vi "LeerBD.vi"(8 "error in (no error)":errorcluster) -> (0 "error out":errorcluster, 2 "BD":T1={"niv_presion_son_ref"=97.0, "Incertidumbre"=["1", "1", "1", "1", "1", "1", "1", "1", "1", "1"], "Tol +"=["2,0", "1,5", "1,5", "1,4", "1,4", "1,1", "1,6", "1,6", "2,1", "3,5"], "Tol -"=["-2,0", "-1,5", "-1,5", "-1,4", "-1,4", "-1,1", "-1,6", "-1,6", "-2,1", "-3,5"], "Frecuencias(Hz)"=["95", "94", "94", "94", "96", "95", "94", "96", "95", "94"]}, 3 "Prueba05 out":refnum<class "Prueba05.lvclass">)   [LabVIEW 2019, in "Prueba05.lvclass"]
uses:
  Prueba05.lvclass
  BD.ctl
  Base de Datos/SQLiteConnector/SQLiteConnection.lvclass
  Base de Datos/Base de Datos.lvclass
panel:
  in  "Tipo Equipo":enum16{"Sonometro", "Calibrador", "Dosimetro"}(ring)
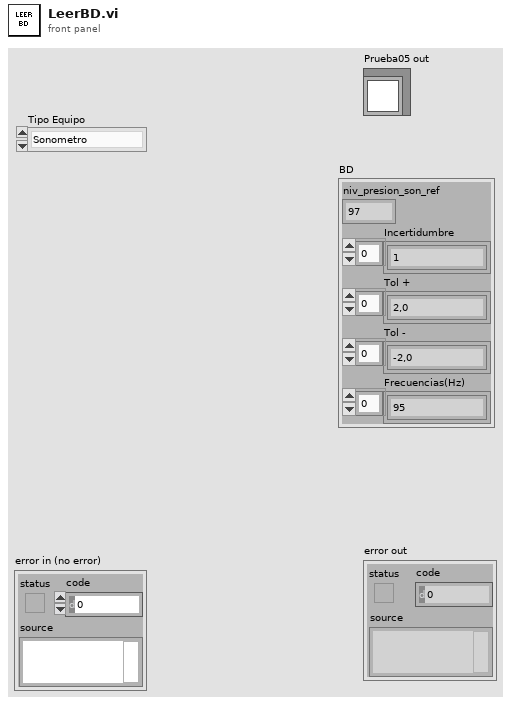
[diagram p1: front panel]
types:
  T1 = typedef "Prueba05.lvclass/BD.ctl" = cluster{"niv_presion_son_ref":dbl, "Incertidumbre":string[], "Tol +":string[], "Tol -":string[], "Frecuencias(Hz)":string[]}
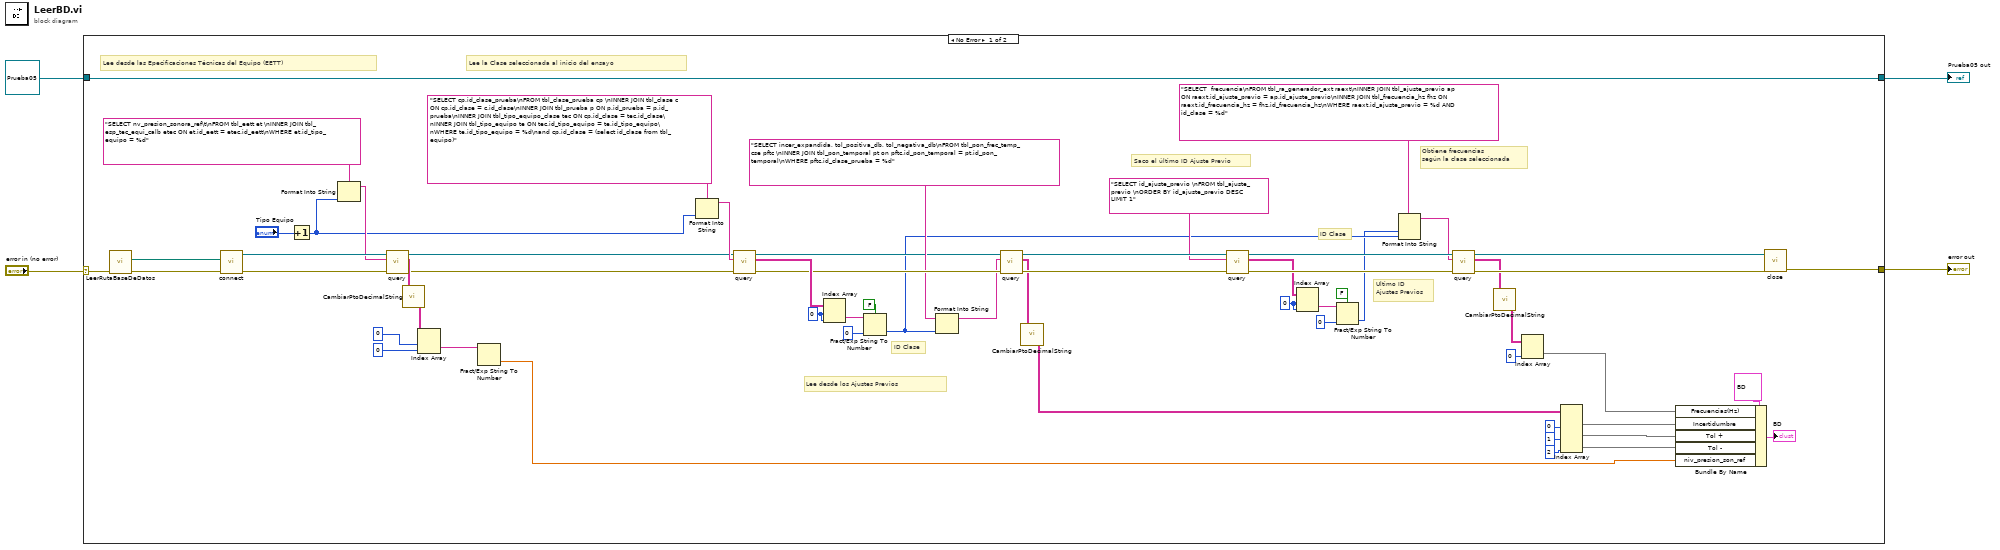
[diagram p0: block diagram]
diagram:
  n1 = case shown="No Error" "error in (no error)" {
    selector: "error in (no error)" -> [w56 w66]
    tunnel: [w42 w66] -> w3
    tunnel: [w64 w65] -> w1
    tunnel: refnum<class "Prueba05.lvclass"> refnum ("Prueba02 in") -> [w64 w65]
    frame No Error {
      w20 = 0 ("index (row)")
      w48 = 0 ("index (row)")
      # "Ultimo ID\nAjustes Previos"
      # "ID Clase"
      # "Obtiene frecuencias\nsegún la clase seleccionada"
      # "ID Clase"
      # "Saco el último ID Ajuste Previo"
      # "Lee desde los Ajustes Previos"
      # "Lee la Clase seleccionada al inicio del ensayo"
      # "Lee desde las Epecificaciones Técnicas del Equipo (EETT)"
      n2 = call "LeerRutaBaseDeDatos.vi"("error in (no error)"=w56) -> ("error out"=w59:errorcluster, "Database Path"=w58:path)  [unwired: 9 in]
      n3 = call "connect.vi"("error in (no error)"=w59, "Database Path"=w58) -> ("error out"=w61:errorcluster, "object out"=w62:refnum<class "SQLiteConnection.lvclass">)  [unwired: 8 in]
      n4 = Increment(x="Tipo Equipo") -> (x+1=w36:enum16{"Sonometro", "Calibrador", "Dosimetro"})
      n5 = Format Into String(format string="SELECT nv_presion_sonora_ref\t\nFROM tbl_eett et \nINNER JOIN tbl_esp_tec_equi_calb etec ON et.id_eett = etec.id_eett\nWHERE et.id_tipo_equipo = %d", w36) -> (resulting string=w60:string)  [unwired: 2 in, 1 out]
      n6 = call "query.vi"("error in (no error)"=w61, "SQL Statement"=w60, "object in"=w62) -> ("error out"=w49:errorcluster, "result"=w53:string[][], "object out"=w50:refnum<class "SQLiteConnection.lvclass">)  [unwired: 5 in, 1 out]
      n7 = call "CambiarPtoDecimalString.vi"("result"=w53) -> ("result out"=w5:string[][])
      n8 = Index Array(array=w5, index (row)=0, index (col)=0 ("disabled index (col)")) -> (element=w54:string)
      n9 = Fract/Exp String To Number(string=w54) -> (number=w10:dbl)  [unwired: 3 in, 1 out]
      n10 = Format Into String(format string="SELECT cp.id_clase_prueba\nFROM tbl_clase_prueba cp \nINNER JOIN tbl_clase c ON cp.id_clase = c.id_clase\nINNER JOIN tbl_prueba p ON p.id_prueba = p.id_prueba\nINNER JOIN tbl_tipo_equipo_clase tec ON cp.id_clase = tec.id_clase\nINNER JOIN tbl_tipo_equipo te ON tec.id_tipo_equipo = te.id_tipo_equipo\nWHERE te.id_tipo_equipo = %d\nand cp.id_clase = (select id_clase from tbl_equipo)", w36) -> (resulting string=w51:string)  [unwired: 2 in, 1 out]
      n11 = call "query.vi"("error in (no error)"=w49, "SQL Statement"=w51, "object in"=w50) -> ("error out"=w43:errorcluster, "result"=w44:string[][], "object out"=w39:refnum<class "SQLiteConnection.lvclass">)  [unwired: 5 in, 1 out]
      n12 = Index Array(array=w44, index (row)=w48, index (col)=w48) -> (element=w46:string)
      n13 = Fract/Exp String To Number(use system decimal point (T)=FALSE, string=w46, default (0 dbl)=0 ("index (row)")) -> (number=w16:i32)  [unwired: 1 in, 1 out]
      n14 = Format Into String(format string="SELECT incer_expandida, tol_positiva_db, tol_negativa_db\nFROM tbl_pon_frec_temp_cse pftc \nINNER JOIN tbl_pon_temporal pt on pftc.id_pon_temporal = pt.id_pon_temporal\nWHERE pftc.id_clase_prueba = %d", w16) -> (resulting string=w38:string)  [unwired: 2 in, 1 out]
      n15 = call "query.vi"("error in (no error)"=w43, "SQL Statement"=w38, "object in"=w39) -> ("error out"=w40:errorcluster, "result"=w31:string[][], "object out"=w26:refnum<class "SQLiteConnection.lvclass">)  [unwired: 5 in, 1 out]
      n16 = call "CambiarPtoDecimalString.vi"("result"=w31) -> ("result out"=w6:string[][])
      n17 = call "query.vi"("error in (no error)"=w40, "SQL Statement"="SELECT id_ajuste_previo \nFROM tbl_ajuste_previo \nORDER BY id_ajuste_previo DESC LIMIT 1" ("format string"), "object in"=w26) -> ("error out"=w27:errorcluster, "result"=w19:string[][], "object out"=w25:refnum<class "SQLiteConnection.lvclass">)  [unwired: 5 in, 1 out]
      n18 = Index Array(array=w19, index (row)=w20, index (col)=w20) -> (element=w22:string)
      n19 = Fract/Exp String To Number(use system decimal point (T)=FALSE, string=w22, default (0 dbl)=0 ("index (row)")) -> (number=w14:i32)  [unwired: 1 in, 1 out]
      n20 = Format Into String(format string="SELECT  frecuencia\nFROM tbl_ra_generador_ext raext\nINNER JOIN tbl_ajuste_previo ap ON raext.id_ajuste_previo = ap.id_ajuste_previo\nINNER JOIN tbl_frecuencia_hz fhz ON raext.id_frecuencia_hz = fhz.id_frecuencia_hz\nWHERE raext.id_ajuste_previo = %d AND id_clase = %d", w14, w16) -> (resulting string=w17:string)  [unwired: 2 in, 1 out]
      n21 = call "query.vi"("error in (no error)"=w27, "SQL Statement"=w17, "object in"=w25) -> ("error out"=w37:errorcluster, "result"=w35:string[][], "object out"=w15:refnum<class "SQLiteConnection.lvclass">)  [unwired: 5 in, 1 out]
      n22 = call "CambiarPtoDecimalString.vi"("result"=w35) -> ("result out"=w7:string[][])
      n23 = Index Array(array=w7, index (col)=0 ("disabled index (col)")) -> (element=w8:string[])  [unwired: 1 in]
      n24 = Index Array(array=w6, index (col) #1=0 ("disabled index (col)"), index (col) #2=1 ("index (col)"), index (col) #3=2 ("index (col)")) -> (element #1=w34:string[], element #2=w33:string[], element #3=w32:string[])  [unwired: 3 in]
      n25 = Bundle By Name(cluster=T1 {"niv_presion_son_ref"=97.0, "Incertidumbre"=["1", "1", "1", "1", "1", "1", "1", "1", "1", "1"], "Tol +"=["2,0", "1,5", "1,5", "1,4", "1,4", "1,1", "1,6", "1,6", "2,1", "3,5"], "Tol -"=["-2,0", "-1,5", "-1,5", "-1,4", "-1,4", "-1,1", "-1,6", "-1,6", "-2,1", "-3,5"], "Frecuencias(Hz)"=["95", "94", "94", "94", "96", "95", "94", "96", "95", "94"]} ("BD"), "Frecuencias(Hz)"=w8, "Incertidumbre"=w34, "Tol +"=w33, "Tol -"=w32, "niv_presion_son_ref"=w10) -> (→"BD":T1)
      n26 = call-dynamic "close.vi"("error in (no error)"=w37, "object in"=w15) -> ("error out"=w42:errorcluster)  [unwired: 8 in, 1 out]
    }
    frame Error {
    }
  }
  "error out" <- w3
  "Prueba05 out" <- w1
